vi "Kinect MVMT.vi"() -> ()   [LabVIEW 2011]
uses:
  <vilib>/Platform/TimedLoop/XDataNode/XDataNode.xnode
  <vilib>/Platform/TimedLoop/XDataNode/nitl_modes.ctl
  <vilib>/Platform/TimedLoop/XDataNode/XDNodeRunTimeDep.lvlib
  <vilib>/Platform/TimedLoop/XDataNode/wakeup.ctl
  <vilib>/Platform/TimedLoop/XDataNode/timing_clust.ctl
  <vilib>/Utility/sysdir.llb/System Directory Type.ctl
  <vilib>/vision/NI_Vision_Development_Module.lvlib
panel:
  in  "Diff Image Thing":i32=5 min=0 max=7
  out "Right - Left (Diff Img)":sgl(graph)
  out "Right - Left (Raw Img)":sgl(graph)
  out "Angle":dbl(graph)
  out "Extracted Difference Contour":T1(plugin-control)
  out "Right Diff":T2(graph)
  out "Left Diff":T2(graph)
  out "Right Raw":T2(graph)
  out "Left Raw":T2(graph)
  out "Difference Image":T1(plugin-control)
  in  "Spline Style":u16(ring)=2 items=["equally spaced", "chord length", "centripetal"]
  in  "# Points in Spline":i32=50
  in  "degree":i32=3
  out "Extracted Contour":T1(plugin-control)
  out "Occupancy Map":T1(plugin-control)
  in  "Number of Openings":i32=3
  in  "Selection Values":T4(array[cluster]) {"Measurement Parameter" items=["Center of Mass X", "Center of Mass Y", "First Pixel X", "First Pixel Y", "Bounding Rect Left", "Bounding Rect Top", "Bounding Rect Right", "Bounding Rect Bottom", "Max Feret Diameter Start X", "Max Feret Diameter Start Y", "Max Feret Diameter End X", "Max Feret Diameter End Y", "Max Horiz. Segment Length Left", "Max Horiz. Segment Length Right", "Max Horiz. Segment Length Row", "-", "Bounding Rect Width", "Bounding Rect Height", "Bounding Rect Diagonal", "Perimeter", "Convex Hull Perimeter", "Holes' Perimeter", "Max Feret Diameter", "Equivalent Ellipse Major Axis", "Equivalent Ellipse Minor Axis", "Equivalent Ellipse Minor Axis (Feret)", "Equivalent Rect Long Side", "Equivalent Rect Short Side", "Equivalent Rect Diagonal", "Equivalent Rect Short Side (Feret)", "Average Horiz. Segment Length", "Average Vert. Segment Length", "Hydraulic Radius", "Waddel Disk Diameter", "-", "Area", "Holes' Area", "Particle & Holes' Area", "Convex Hull Area", "Image Area", "-", "Number of Holes", "Number of Horiz. Segments", "Number of Vert. Segments", "-", "Orientation", "Max Feret Diameter Orientation", "-", "% Area/Image Area", "% Area/(Particle & Holes' Area)", "Ratio of Equivalent Ellipse Axes", "Ratio of Equivalent Rect Sides", "-", "Elongation Factor", "Compactness Factor", "Heywood Circularity Factor", "Type Factor", "-", "Sum X", "Sum Y", "Sum XX", "Sum XY", "Sum YY", "Sum XXX", "Sum XXY", "Sum XYY", "Sum YYY", "-", "Moment of Inertia XX", "Moment of Inertia XY", "Moment of Inertia YY", "Moment of Inertia XXX", "Moment of Inertia XXY", "Moment of Inertia XYY", "Moment of Inertia YYY", "Norm. Moment of Inertia XX", "Norm. Moment of Inertia XY", "Norm. Moment of Inertia YY", "Norm. Moment of Inertia XXX", "Norm. Moment of Inertia XXY", "Norm. Moment of Inertia XYY", "Norm. Moment of Inertia YYY", "Hu Moment 1", "Hu Moment 2", "Hu Moment 3", "Hu Moment 4", "Hu Moment 5", "Hu Moment 6", "Hu Moment 7"]; "Range Lower Value" format="%.2f"; "Range Upper Value" format="%.2f"}
  in  "Contour Length Threshold":dbl(slide)=126.92307692307692 min=-32768.0 max=32768.0 step=1.0 scale=0.0..500.0
  in  "Display Type":T5(ring)=enum."Baseline Extracted"
  in  "Post Extraction Limit":cluster{dbl, dbl}(slide)={48.0, 888.0} scale=-3000.0..3000.0
  in  "stop 2":bool
  in  "# Frames in Average":i32=100
  in  "Start":bool
  in  "Zero Out Baseline":bool
  in  "Median Filter Size":i32=5 min=0 max=7
  in  "Divisor":sgl=0.5 min=0 max=1 step=0.1
  in  "Name or Relative Path":string="Mouse Test"
  in  "Distance to Camera Visible":cluster{dbl, dbl}(slide)={-4718.592, 13369.344000000001} scale=-32768.0..32768.0
  in  "Status":string
  out "Frame Display":T1(plugin-control)
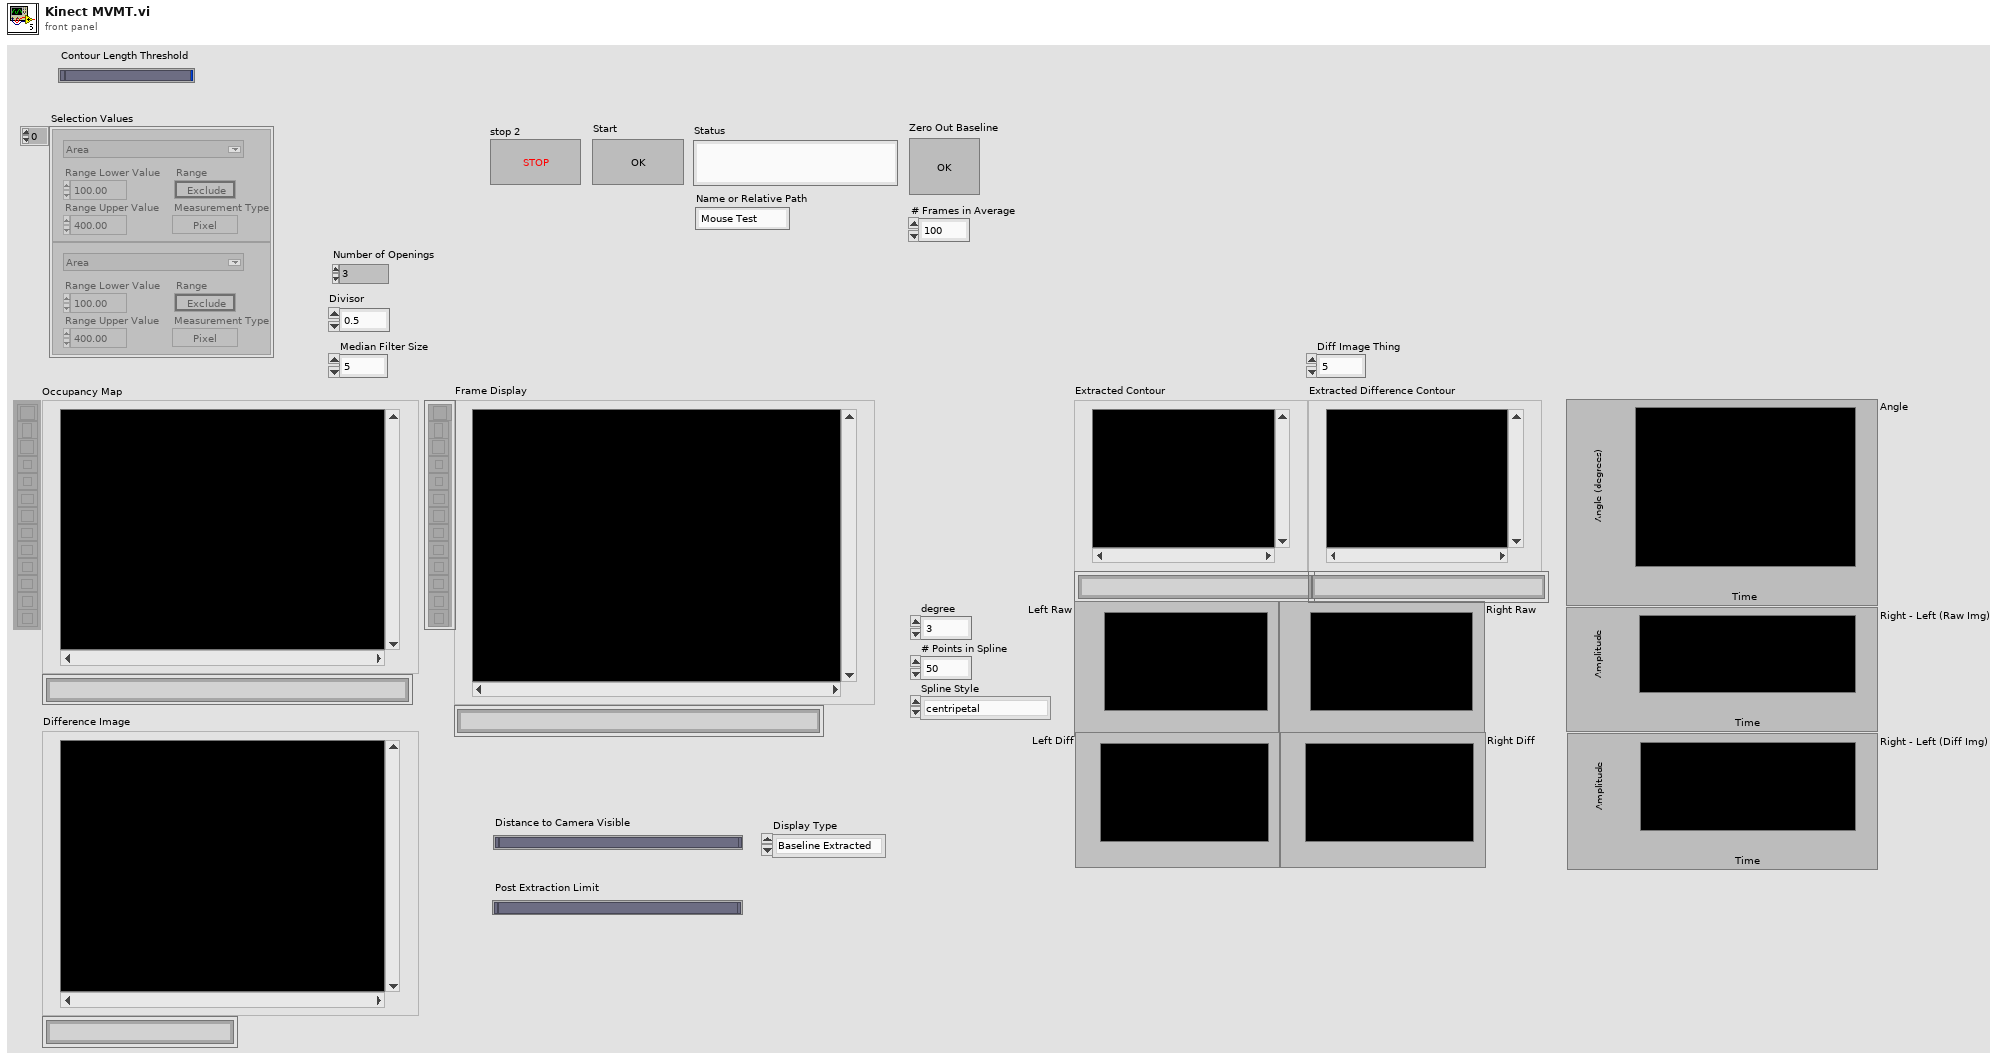
[diagram p1: front panel]
types:
  T1 = typedef "IMAQ Image.ctl" = refnum<image>
  T2 = cluster{"Starting Value":sgl, "Incremental Value":sgl, "Histogram":u32[]}
  T3 = typedef "Particle Parameters" = i32
  T4 = cluster{"Measurement Parameter":T3, "Range Lower Value":dbl, "Range Upper Value":dbl, "Range":bool, "Measurement Type":bool}[]
  T5 = enum16{"Raw Image", "Baseline", "Baseline Extracted"}
  T6 = typedef "Image Type" = u32
  T7 = typedef "System Directory Type.ctl" = i32
  T8 = enum16{"Record", "Idle", "Acquire Background", "Stop"}
  T9 = typedef "XDNodeRunTimeDep.lvlib/timing_clust.ctl" = cluster{"Expected End [f-1]":u64, "Actual End [f-1]":u64, "Finished Late? [f-1]":bool, "Expected End [i-1]":u64, "Actual End [i-1]":u64, "Finished Late? [i-1]":bool, "Expected Start [i]":u64, "Actual Start [i]":u64, "Expected Start [f]":u64, "Actual Start [f]":u64, "Source Name":string, "Structure Name":string, "Period":i64, "Deadline":i64, "Offset":i64, "Start":i64, "Priority":i32, "Timeout":i32, "Mode":T10, "Wakeup Reason":T11, "Error":errorcluster, "Source Type":string, "Secondary Source Type":string, "Global End Time":u64, "Global Start Time":u64, "Frame Duration":u64, "Iteration Duration":u64, "Assigned CPU":i32, "I/O Scan Engine Mode":u32}
  T10 = typedef "XDNodeRunTimeDep.lvlib/nitl_modes.ctl" = enum32{"No Change", "Process missed periods, maintain original phase", "Discard missed periods, maintain original phase", "Process missed periods, ignore original phase", "Discard missed periods, ignore original phase"}
  T11 = typedef "XDNodeRunTimeDep.lvlib/wakeup.ctl" = enum32{"Normal", "Aborted", "Asynchronous wakeup", "Timing source error", "Timed loop error", "Timeout"}
  T12 = enum32{"Average", "Min", "Max", "Clear  if < ", "Clear  if < or =", "Clear  if =", "Clear  if > or =", "Clear  if >"}
  T13 = cluster{"Median Filter Size":i32, "Median Filter Size":i32, i32}
  T14 = cluster{"Area":dbl, "Number of Holes":dbl, "Bounding Rect":cluster{"Left":dbl, "Top":dbl, "Right":dbl, "Bottom":dbl}, "Center of Mass":cluster{"X":dbl, "Y":dbl}, "Orientation":dbl, "Dimensions":cluster{"Width":dbl, "Height":dbl}}[]
  T15 = typedef "ROI Descriptor" = cluster{"Global Rectangle":i32[], "Contours":cluster{"ID":enum32{"External", "Internal"}, "Type":u32, "Coordinates":i32[]}[]}
  T16 = cluster{"Area":dbl, "Number of Holes":dbl, "Bounding Rect":cluster{"Left":dbl, "Top":dbl, "Right":dbl, "Bottom":dbl}, "Center of Mass":cluster{"X":dbl, "Y":dbl}, "Orientation":dbl, "Dimensions":cluster{"Width":dbl, "Height":dbl}}
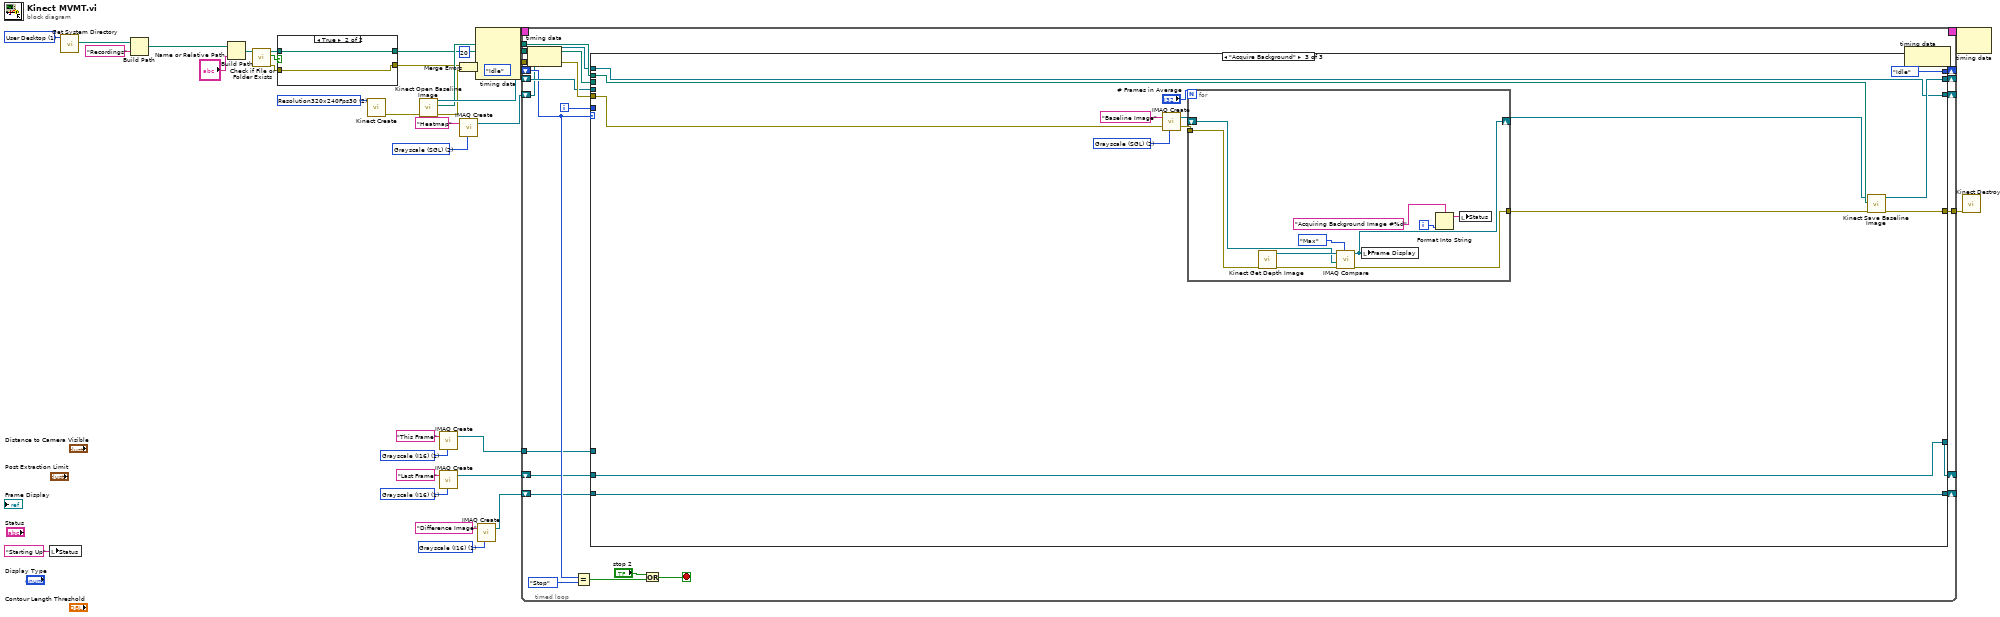
[diagram p0: block diagram]
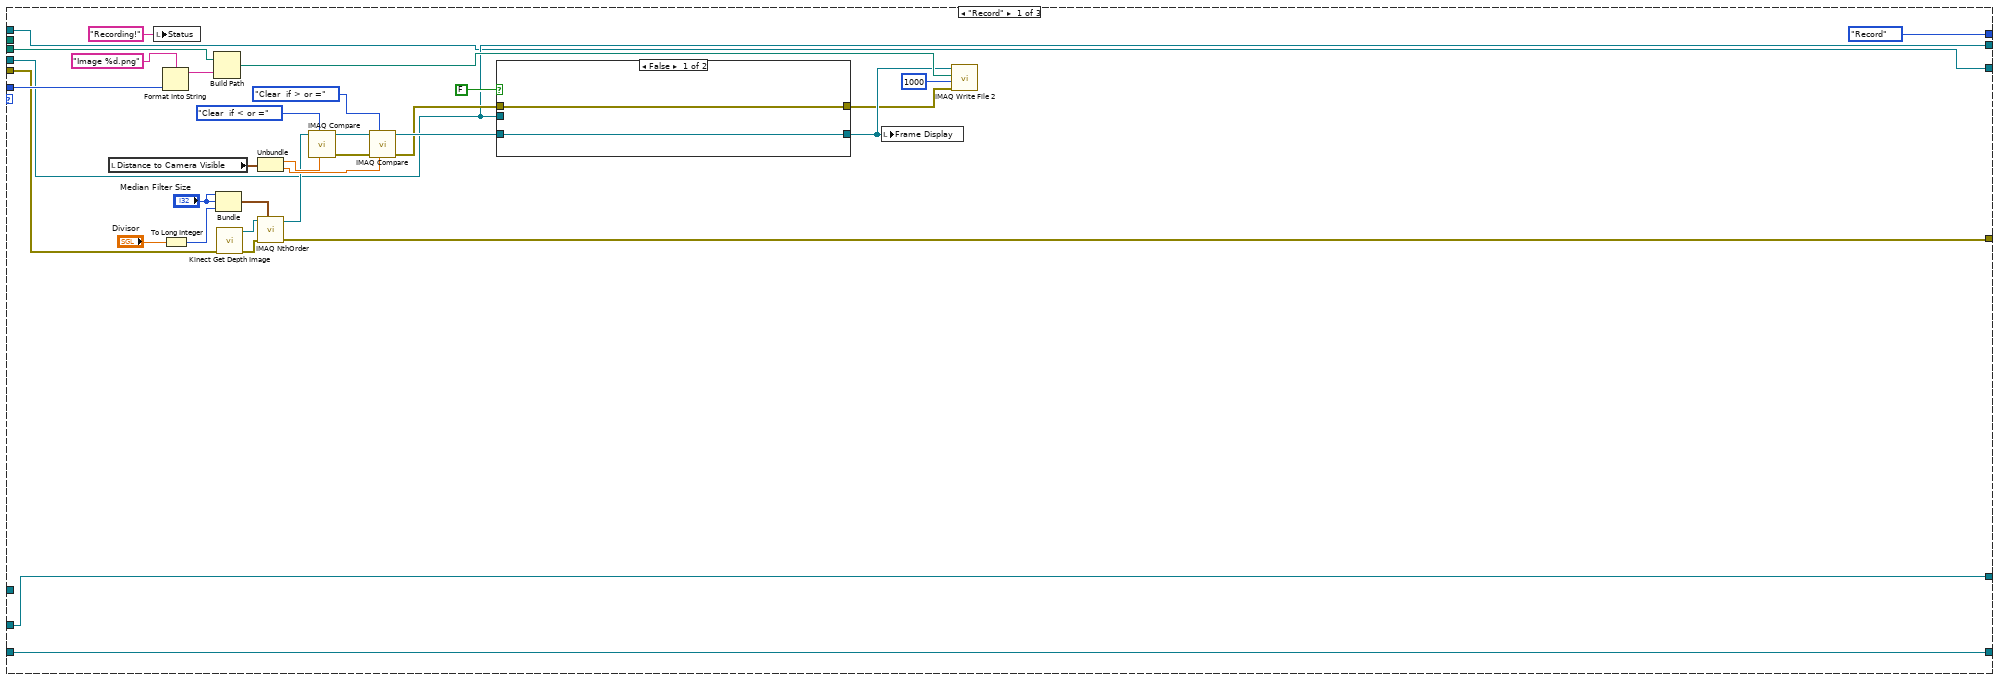
[diagram p2: hidden frame]
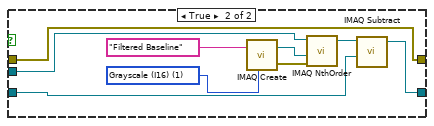
[diagram p3: hidden frame]
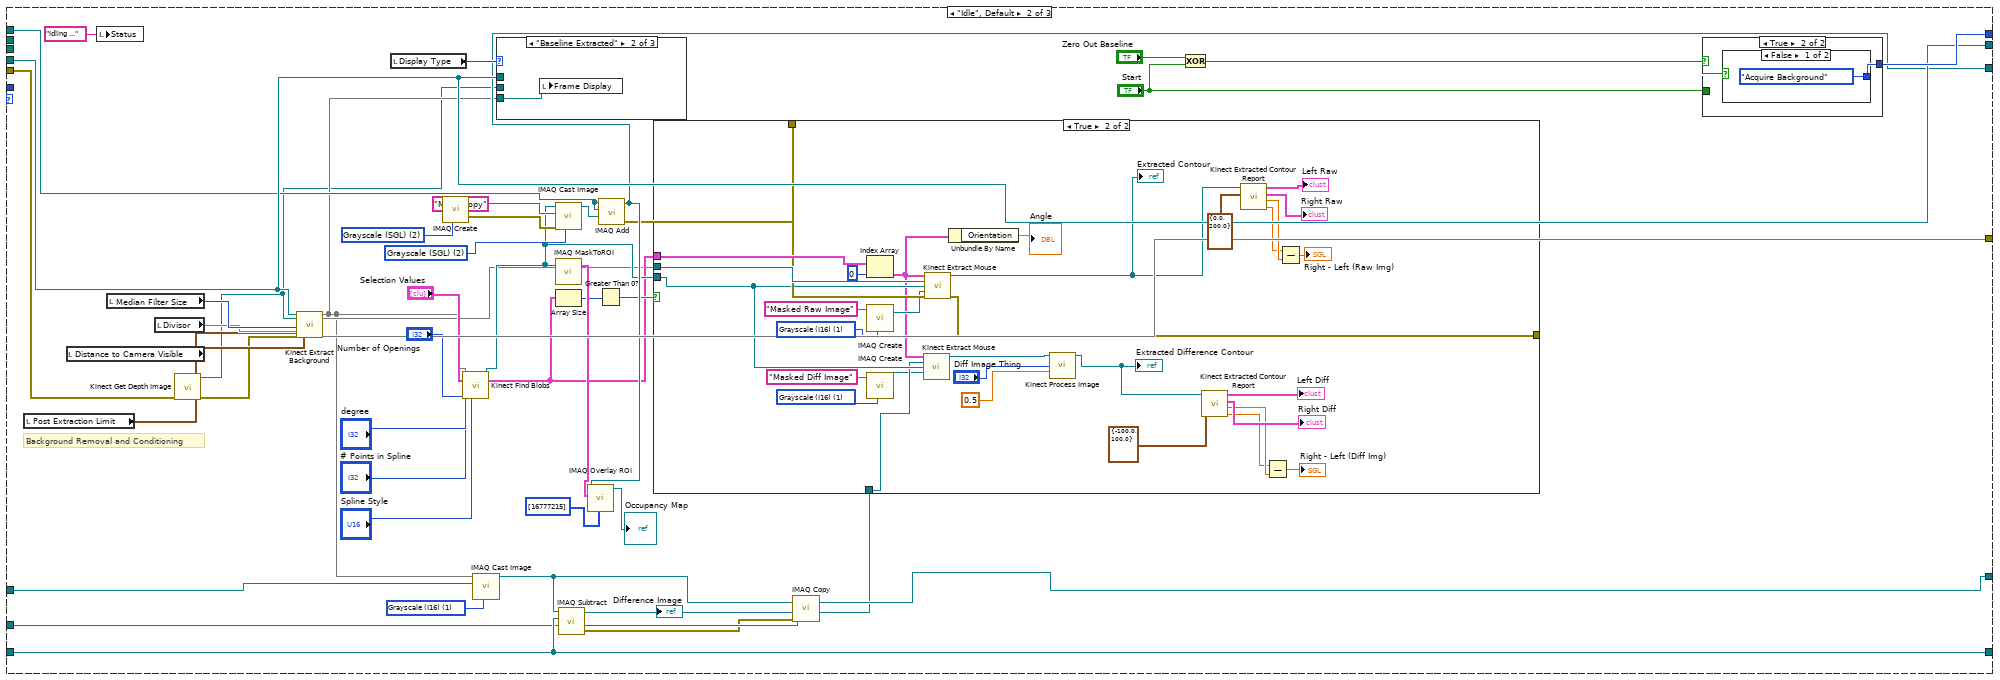
[diagram p4: hidden frame]
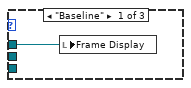
[diagram p6: hidden frame]
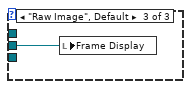
[diagram p7: hidden frame]
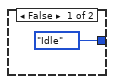
[diagram p8: hidden frame]
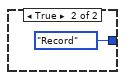
[diagram p9: hidden frame]
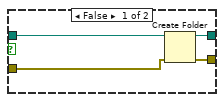
[diagram p10: hidden frame]
diagram:
  w2 = T6 1 items=["Grayscale (U8)", "Grayscale (I16)", "Grayscale (SGL)", "Complex (CSG)", "RGB (U32)", "HSL (U32)", "RGB (U64)", "Grayscale (U16)"] ("Image Type")
  w6 = T6 1 items=["Grayscale (U8)", "Grayscale (I16)", "Grayscale (SGL)", "Complex (CSG)", "RGB (U32)", "HSL (U32)", "RGB (U64)", "Grayscale (U16)"] ("Image Type")
  w9 = T6 1 items=["Grayscale (U8)", "Grayscale (I16)", "Grayscale (SGL)", "Complex (CSG)", "RGB (U32)", "HSL (U32)", "RGB (U64)", "Grayscale (U16)"] ("Image Type")
  w15 = T6 2 items=["Grayscale (U8)", "Grayscale (I16)", "Grayscale (SGL)", "Complex (CSG)", "RGB (U32)", "HSL (U32)", "RGB (U64)", "Grayscale (U16)"] ("Image Type")
  w31 = 2 items=["Undefined", "Resolution640x480Fps30", "Resolution320x240Fps30", "Resolution80x60Fps30"] ("Depth Format")
  w33 = T7 1 items=["User Home"=0, "User Desktop"=1, "User Documents"=2, "User Application Data"=3, "User Preferences"=4, "User Temporary"=5, "Public Documents"=6, "Public Application Data"=7, "Public Preferences"=8, "Public Cache"=13, "System Core Libraries"=9, "System Installed Libraries"=10, "Application Files"=11, "Boot Volume Root"=12] ("system directory type")
  n1 = local write "Status"("Starting Up" ("Status")) -> ()
  n2 = call <vilib>:"Get System Directory.vi"("system directory type"=w33) -> ("system directory"=w32:path)  [unwired: 10 in]
  n3 = Build Path(base path=w32, name or relative path="Recordings") -> (appended path=w26:path)
  n4 = Build Path(base path=w26, name or relative path="Name or Relative Path") -> (appended path=w17:path)
  n5 = call <vilib>:"Check if File or Folder Exists.vi"("path"=w17) -> ("error out"=w24:errorcluster, "file or folder exists?"=w22:bool, "dup path"=w23:path)  [unwired: 8 in]
  n6 = case shown="True" w22 {
    tunnel: w24 -> [w39 w40]
    tunnel: w23 -> [w38 w41]
    tunnel: [w36 w41] -> w21
    tunnel: [w37 w40] -> w18
    frame False {
      n7 = Create Folder(path (use dialog)=w38, error in=w39) -> (created path=w36:path, error out=w37:errorcluster)  [unwired: 1 in, 1 out]
    }
    frame True {
    }
  }
  n8 = call "Kinect Create.vi"("Depth Format"=w31) -> ("error out"=w28:errorcluster)  [unwired: 9 in, 1 out]
  n9 = call "Kinect Open Baseline Image.vi"("error in (no error)"=w28) -> ("error out"=w19:errorcluster, "Background Image Path"=w29:path, "Background Image"=w30:T1)  [unwired: 8 in]
  n10 = call "IMAQ Create"("Image Name"="This Frame", "Image Type"=w6) -> ("New Image"=w4:T1)  [unwired: 3 in, 1 out]
  n11 = call "IMAQ Create"("Image Name"="Last Frame", "Image Type"=w9) -> ("New Image"=w7:T1)  [unwired: 3 in, 1 out]
  n12 = Merge Errors(w18, w19) -> (w20:errorcluster)
  n13 = call "IMAQ Create"("Image Name"="Heatmap", "Image Type"=w15) -> ("New Image"=w13:T1)  [unwired: 3 in, 1 out]
  n14 = node-c288(i64 20 ("Period")) -> (w12:T9)  [unwired: 3 in]
  n15 = call "IMAQ Create"("Image Name"="Difference Image", "Image Type"=w2) -> ("New Image"=w1:T1)  [unwired: 3 in, 1 out]
  n16 = timed-loop {
    tunnel: w20 -> [w61]
    tunnel: [w60] -> w16
    shift-right: [w53] -> _
    shift-left: T8."Idle" -> [w55]
    shift-right: [w52] -> _
    shift-left: w30 -> [w59]
    tunnel: w29 -> [w51]
    tunnel: w21 -> [w49]
    shift-right: [w47] -> _
    shift-left: w13 -> [w48]
    timing: w12 -> [_]
    timing-out: [_] -> w11
    shift-right: [w46] -> _
    shift-left: w7 -> [w45]
    tunnel: w4 -> [w44]
    shift-right: [w42] -> _
    shift-left: w1 -> [w43]
    i -> [w50]
    stop <- w57 stop-if-true
    n17 = node-c288() -> ()  [unwired: 1 in, 1 out]
    n18 = Equal?(x=w55, y=T8."Stop") -> (x = y?=w56:bool)
    n19 = case shown="\"Acquire Background\"" w55 {
      tunnel: w61 -> [w76 w148 w205]
      tunnel: [w85 w144 w201] -> w60
      tunnel: w59 -> [w67 w142 _]
      tunnel: [T8."Record" w149 T8."Idle"] -> w53
      tunnel: [w67 w142 w202] -> w52
      tunnel: w51 -> [_ _ w199]
      tunnel: w50 -> [w82 _ _]
      tunnel: w49 -> [w81 _ _]
      tunnel: w48 -> [w66 w129 w197]
      tunnel: [w66 w138 w197] -> w47
      tunnel: w45 -> [w65 w114 w196]
      tunnel: [w65 w112 w196] -> w46
      tunnel: w44 -> [_ w118 _]
      tunnel: w43 -> [w64 w115 w195]
      tunnel: [w64 w115 w195] -> w42
      frame "Record" {
        n20 = local read "Distance to Camera Visible"() -> (w88:cluster{dbl, dbl})
        n21 = local write "Status"("Recording!" ("Status")) -> ()
        n22 = Format Into String(format string="Image %d.png", w82) -> (resulting string=w83:string)  [unwired: 2 in, 1 out]
        n23 = To Long Integer(number="Divisor") -> (32bit integer=w87:i32)
        n24 = Build Path(base path=w81, name or relative path=w83) -> (appended path=w80:path)
        n25 = Bundle("Median Filter Size"="Median Filter Size", "Median Filter Size"="Median Filter Size", w87) -> (w74:T13)  [unwired: 1 in]
        n26 = call "Kinect Get Depth Image.vi"("error in (no error)"=w76) -> ("error out"=w77:errorcluster, "Depth Image"=w75:T1)  [unwired: 9 in]
        n27 = Unbundle(w88) -> (w91:dbl, w90:dbl)
        n28 = call "IMAQ NthOrder"("Image Src"=w75, "Size & Order #"=w74, "error in (no error)"=w77) -> ("Image Dst Out"=w73:T1, "error out"=w85:errorcluster)  [unwired: 4 in]
        n29 = call "IMAQ Compare"("Constant"=w91, "Operator"=T12."Clear  if < or =", "Image Src A"=w73) -> ("error out"=w93:errorcluster, "Image Dst Out"=w92:T1)  [unwired: 7 in]
        n30 = call "IMAQ Compare"("Constant"=w90, "Operator"=T12."Clear  if > or =", "error in (no error)"=w93, "Image Src A"=w92) -> ("error out"=w70:errorcluster, "Image Dst Out"=w72:T1)  [unwired: 6 in]
        n31 = case shown="False" FALSE {
          tunnel: w72 -> [w98 w99]
          tunnel: [w98 w107] -> w71
          tunnel: [w97 w106] -> w69
          tunnel: w70 -> [w97 w106]
          tunnel: w67 -> [_ w101]
          frame False {
          }
          frame True {
            w105 = T6 1 items=["Grayscale (U8)", "Grayscale (I16)", "Grayscale (SGL)", "Complex (CSG)", "RGB (U32)", "HSL (U32)", "RGB (U64)", "Grayscale (U16)"] ("Image Type")
            n32 = call "IMAQ Create"("Image Name"="Filtered Baseline", "Image Type"=w105) -> ("New Image"=w103:T1, "error out"=w102:errorcluster)  [unwired: 3 in]
            n33 = call "IMAQ NthOrder"("Image Src"=w101, "Image Dst"=w103, "error in (no error)"=w102) -> ("Image Dst Out"=w100:T1)  [unwired: 4 in, 1 out]
            n34 = call "IMAQ Subtract"("Image Src A"=w100, "Image Src B"=w99) -> ("Image Dst Out"=w107:T1)  [unwired: 5 in, 1 out]
          }
        }
        n35 = local write "Frame Display"(w71) -> ()
        n36 = call-poly "IMAQ Write File 2"("error in (no error)"=w69, "Image Quality"=u32 1000, "File Path"=w80, "Image"=w71) -> ()  [unwired: 6 in, 2 out]
      }
      frame "Idle", Default {
        w117 = T6 1 items=["Grayscale (U8)", "Grayscale (I16)", "Grayscale (SGL)", "Complex (CSG)", "RGB (U32)", "HSL (U32)", "RGB (U64)", "Grayscale (U16)"] ("Image Type")
        w131 = T6 2 items=["Grayscale (U8)", "Grayscale (I16)", "Grayscale (SGL)", "Complex (CSG)", "RGB (U32)", "HSL (U32)", "RGB (U64)", "Grayscale (U16)"] ("Image Type")
        w136 = T6 2 items=["Grayscale (U8)", "Grayscale (I16)", "Grayscale (SGL)", "Complex (CSG)", "RGB (U32)", "HSL (U32)", "RGB (U64)", "Grayscale (U16)"] ("Image Type")
        # "Background Removal and Conditioning"
        n37 = local read "Post Extraction Limit"() -> (w143:cluster{dbl, dbl})
        n38 = local read "Distance to Camera Visible"() -> (w145:cluster{dbl, dbl})
        n39 = local write "Status"("Idling ..." ("Status")) -> ()
        n40 = local read "Median Filter Size"() -> (w147:i32)
        n41 = local read "Divisor"() -> (w146:sgl)
        n42 = call "Kinect Get Depth Image.vi"("error in (no error)"=w148) -> ("error out"=w108:errorcluster, "Depth Image"=w116:T1)  [unwired: 9 in]
        n43 = call "Kinect Extract Background.vi"(0:w142, 1:w116, 3:w147, 4:w146, 5:w108, 7:w145, 11:w143) -> (14:w119, 15:w120, 19:w144)  [unwired: 10 in]
        n44 = local read "Display Type"() -> (w141:T5)
        n45 = call "IMAQ Create"("Image Name"="Mask Copy", "Image Type"=w136) -> ("New Image"=w133:T1, "error out"=w134:errorcluster)  [unwired: 3 in]
        n46 = call "Kinect Find Blobs.vi"("Image Src"=w119, "Selection Values"="Selection Values", "Number of Erosion"="# Points in Spline", "Range"="degree", "error in"="Number of Openings", 12:"Spline Style") -> ("Masked Image Out"=w128:T1, "Particle Reports (Pixels)"=w124:T14)  [unwired: 6 in, 2 out]
        n47 = call "IMAQ Cast Image"("Image Type"=w117, "Image Dst"=w118, "Image Src"=w119) -> ("Image Dst Out"=w113:T1)  [unwired: 7 in, 1 out]
        n48 = case shown="\"Baseline Extracted\"" w141 {
          tunnel: w119 -> [_ w188 _]
          tunnel: w142 -> [w187 _ _]
          tunnel: w116 -> [_ _ w189]
          frame "Baseline" {
            n49 = local write "Frame Display"(w187) -> ()
          }
          frame "Baseline Extracted" {
            n50 = local write "Frame Display"(w188) -> ()
          }
          frame "Raw Image", Default {
            n51 = local write "Frame Display"(w189) -> ()
          }
        }
        n52 = call "IMAQ Cast Image"("Image Type"=w131, "error in (no error)"=w134, "Image Dst"=w133, "Image Src"=w128) -> ("Image Dst Out"=w132:T1)  [unwired: 6 in, 1 out]
        n53 = call "IMAQ MaskToROI"("Image"=w128) -> ("ROI Descriptor"=w127:T15)  [unwired: 6 in, 2 out]
        n54 = Array Size(array=w124) -> (size(s)=w126:i32)
        n55 = call "IMAQ Subtract"("Image Src A"=w113, "Image Dst"=w115, "Image Src B"=w114) -> ("Image Dst Out"=w109:T1, "error out"=w111:errorcluster)  [unwired: 4 in]
        "Difference Image" <- w109
        n56 = Greater Than 0?(x=w126) -> (x > 0?=w125:bool)
        n57 = call "IMAQ Add"("Image Src A"=w129, "Image Dst"=w129, "Image Src B"=w132) -> ("Image Dst Out"=w138:T1, "error out"=w110:errorcluster)  [unwired: 4 in]
        n58 = call "IMAQ Overlay ROI"("Colors (Green)"=u32[] [16777215], "ROI Descriptor"=w127, "Image"=w138) -> ("Image Out"=→"Occupancy Map":T1)  [unwired: 7 in, 1 out]
        n59 = case shown="True" w125 {
          tunnel: w120 -> [_ w184]
          tunnel: w128 -> [_ w181]
          tunnel: w124 -> [_ w186]
          tunnel: w110 -> [w154 w183]
          tunnel: [w154 w182] -> _
          tunnel: w109 -> [_ w180]
          frame False {
          }
          frame True {
            w176 = T6 1 items=["Grayscale (U8)", "Grayscale (I16)", "Grayscale (SGL)", "Complex (CSG)", "RGB (U32)", "HSL (U32)", "RGB (U64)", "Grayscale (U16)"] ("Image Type")
            w179 = T6 1 items=["Grayscale (U8)", "Grayscale (I16)", "Grayscale (SGL)", "Complex (CSG)", "RGB (U32)", "HSL (U32)", "RGB (U64)", "Grayscale (U16)"] ("Image Type")
            n60 = Index Array(array=w186, index=0) -> (element=w173:T16)
            n61 = call "IMAQ Create"("Image Name"="Masked Raw Image", "Image Type"=w179) -> ("New Image"=w174:T1)  [unwired: 3 in, 1 out]
            n62 = call "IMAQ Create"("Image Name"="Masked Diff Image", "Image Type"=w176) -> ("New Image"=w175:T1)  [unwired: 3 in, 1 out]
            n63 = call "Kinect Extract Mouse.vi"("Particle Report"=w173, "Image Src"=w180, "Image Mask"=w181, "Image Dst"=w175) -> ("Cropped Image Out"=w158:T1)  [unwired: 10 in, 1 out]
            n64 = call "Kinect Extract Mouse.vi"("Particle Report"=w173, "Image Src"=w184, "Image Mask"=w181, "Image Dst"=w174, "error in (no error)"=w183) -> ("Cropped Image Out"=w170:T1, "error out"=w182:errorcluster)  [unwired: 9 in]
            "Extracted Contour" <- w170
            n65 = Unbundle By Name(w173) -> ("Orientation"=→"Angle":dbl)
            n66 = call "Kinect Process Image.vi"("Depth Image In"=w158, "Median Filter Size"="Diff Image Thing", "Divisor"=sgl 0.5) -> ("Image Dst Out"=w155:T1)  [unwired: 11 in, 1 out]
            "Extracted Difference Contour" <- w155
            n67 = call "Kinect Extracted Contour Report.vi"("Interval Range"=cluster{"Minimum":sgl, "Maximum":sgl} {"Minimum"=-100.0, "Maximum"=100.0}, "Image"=w155) -> ("Mean Right Value"=w160:sgl, "Mean Left Value"=w161:sgl, "Right Histogram"=→"Right Diff":T2, "Left Histogram"=→"Left Diff":T2)  [unwired: 6 in]
            n68 = call "Kinect Extracted Contour Report.vi"("Interval Range"=cluster{"Minimum":sgl, "Maximum":sgl} {"Minimum"=0.0, "Maximum"=200.0}, "Image"=w170) -> ("Mean Right Value"=w163:sgl, "Mean Left Value"=w164:sgl, "Right Histogram"=→"Right Raw":T2, "Left Histogram"=→"Left Raw":T2)  [unwired: 6 in]
            n69 = Subtract(x=w160, y=w161) -> (x-y=→"Right - Left (Diff Img)":sgl)
            n70 = Subtract(x=w163, y=w164) -> (x-y=→"Right - Left (Raw Img)":sgl)
          }
        }
        n71 = call "IMAQ Copy"("error in (no error)"=w111, "Image Dst"=w114, "Image Src"=w113) -> ("Image Dst Out"=w112:T1)  [unwired: 3 in, 1 out]
        n72 = Exclusive Or(1:"Start", 2:"Zero Out Baseline") -> (0:w151:bool)
        n73 = case shown="True" w151 {
          tunnel: "Start" -> [_ w192]
          tunnel: [T8."Idle" w191] -> w149
          frame False {
          }
          frame True {
            n74 = case shown="False" w192 {
              tunnel: [T8."Acquire Background" T8."Record"] -> w191
              frame False {
              }
              frame True {
              }
            }
          }
        }
      }
      frame "Acquire Background" {
        w208 = T6 2 items=["Grayscale (U8)", "Grayscale (I16)", "Grayscale (SGL)", "Complex (CSG)", "RGB (U32)", "HSL (U32)", "RGB (U64)", "Grayscale (U16)"] ("Image Type")
        n75 = call "IMAQ Create"("Image Name"="Baseline Image", "Image Type"=w208, "error in (no error)"=w205) -> ("New Image"=w207:T1, "error out"=w204:errorcluster)  [unwired: 2 in]
        n76 = for {
          N: "# Frames in Average" -> [_]
          tunnel: w204 -> [w216]
          shift-right: [w210] -> w198
          shift-left: w207 -> [w213]
          tunnel: [w211] -> w200
          i -> [w217]
          n77 = call "Kinect Get Depth Image.vi"("error in (no error)"=w216) -> ("error out"=w212:errorcluster, "Depth Image"=w214:T1)  [unwired: 9 in]
          n78 = call "IMAQ Compare"("Operator"=T12."Max", "error in (no error)"=w212, "Image Src B"=w213, "Image Src A"=w214) -> ("error out"=w211:errorcluster, "Image Dst Out"=w210:T1)  [unwired: 6 in]
          n79 = local write "Frame Display"(w210) -> ()
          n80 = Format Into String(format string="Acquiring Background Image #%d" ("Status"), w217) -> (resulting string=w219:string)  [unwired: 2 in, 1 out]
          n81 = local write "Status"(w219) -> ()
        }
        n82 = call "Kinect Save Baseline Image.vi"("error in (no error)"=w200, "Baseline Image Path"=w199, "Baseline Image"=w198) -> ("error out"=w201:errorcluster, "Baseline Image Out"=w202:T1)  [unwired: 7 in]
      }
    }
    n83 = Or(x="stop 2", y=w56) -> (x .or. y?=w57:bool)
    n84 = node-c288() -> ()  [unwired: 1 in, 1 out]
  }
  n85 = node-c288(w11) -> ()  [unwired: 1 out]
  n86 = call "Kinect Destroy.vi"("error in"=w16) -> ()  [unwired: 10 in, 1 out]
